vi "AppConfigTypeToXML.vi"(8 "error in (no error)":errorcluster, 11 "RingdownPlugin in":refnum<class "RingdownPlugin.lvclass">) -> (0 "error out":errorcluster, 2 "ConfigXML out":string, 3 "RingdownPlugin out":refnum<class "RingdownPlugin.lvclass">)   [LabVIEW 2014, in "AppPlugins.lvlib" / "RingdownPlugin.lvclass"]
uses:
  RingdownPlugin.lvclass
  RingdownPlugin.lvclass/RingdownPlugin.ctl
  Accessors/Read RingdownConfig.vi
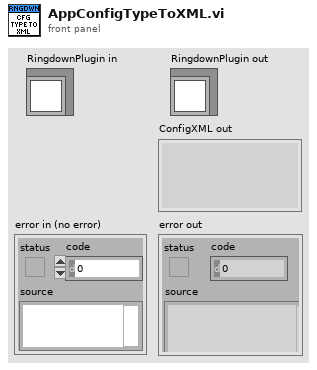
[diagram p1: front panel]
types:
  T1 = typedef "AppPlugins.lvlib/RingdownPlugin.lvclass/RingdownConfig.ctl" = cluster{"Config":cluster{"Addmod":i32, "Scalmod":i32, "Lpocon":i32, "Pircon":i32, "Dmodes":i32, "Lpmcon":u16, "Lpacon":u16, "Fbcon":u16, "Ordcon":i32, "Trimre":dbl, "Ftrimh":dbl, "Ftriml":dbl}, "Window":cluster{"StOffset":i32, "EndOffset":i32, "Length":i32}, "V index":i32, "I index":i32, "PosSeq":bool}
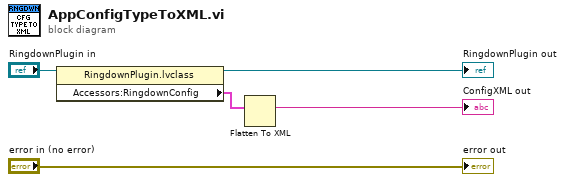
[diagram p0: block diagram]
diagram:
  n1 = property class="RingdownPlugin.lvclass"(reference="RingdownPlugin in") -> (reference out=→"RingdownPlugin out":refnum<class "RingdownPlugin.lvclass">, "Accessors:RingdownConfig"=w4:T1)  [unwired: 1 in, 1 out]
  n2 = Flatten To XML(anything=w4) -> (xml string=→"ConfigXML out":string)
  "error out" <- "error in (no error)"
